vi "精度表.vi"() -> (2 "精度":i32[](array[numeric]), 3 "参数":string[](array[string]))   [LabVIEW 2016, in "数据查询.lvlib"]
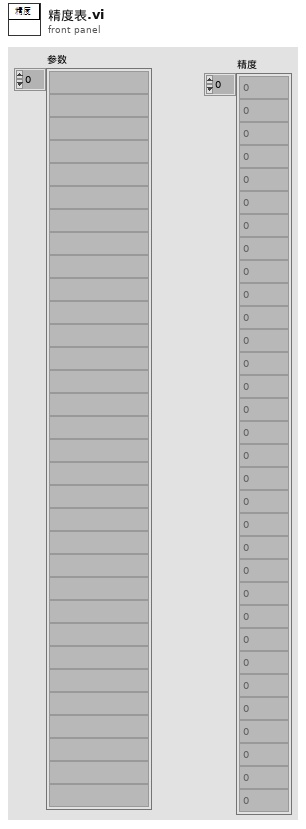
[diagram p1: front panel]
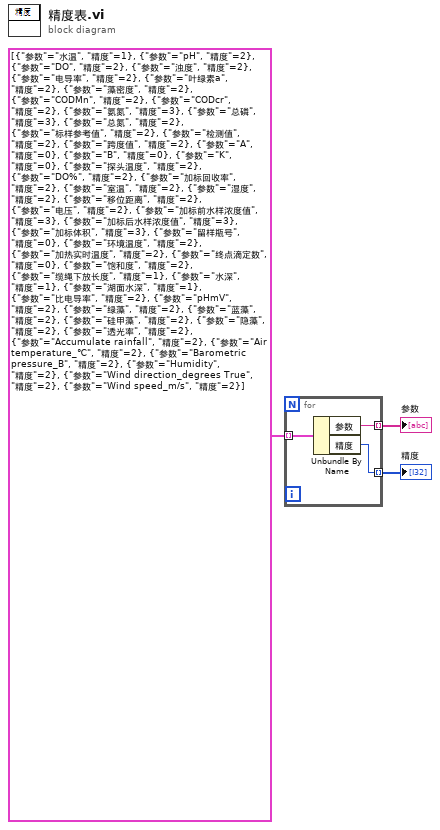
[diagram p0: block diagram]
diagram:
  n1 = for {
    tunnel: cluster{"参数":string, "精度":i32}[] [{"参数"="水温", "精度"=1}, {"参数"="pH", "精度"=2}, {"参数"="DO", "精度"=2}, {"参数"="浊度", "精度"=2}, {"参数"="电导率", "精度"=2}, {"参数"="叶绿素a", "精度"=2}, {"参数"="藻密度", "精度"=2}, {"参数"="CODMn", "精度"=2}, {"参数"="CODcr", "精度"=2}, {"参数"="氨氮", "精度"=3}, {"参数"="总磷", "精度"=3}, {"参数"="总氮", "精度"=2}, {"参数"="标样参考值", "精度"=2}, {"参数"="检测值", "精度"=2}, {"参数"="跨度值", "精度"=2}, {"参数"="A", "精度"=0}, {"参数"="B", "精度"=0}, {"参数"="K", "精度"=0}, {"参数"="探头温度", "精度"=2}, {"参数"="DO%", "精度"=2}, {"参数"="加标回收率", "精度"=2}, {"参数"="室温", "精度"=2}, {"参数"="湿度", "精度"=2}, {"参数"="移位距离", "精度"=2}, {"参数"="电压", "精度"=2}, {"参数"="加标前水样浓度值", "精度"=3}, {"参数"="加标后水样浓度值", "精度"=3}, {"参数"="加标体积", "精度"=3}, {"参数"="留样瓶号", "精度"=0}, {"参数"="环境温度", "精度"=2}, {"参数"="加热实时温度", "精度"=2}, {"参数"="终点滴定数", "精度"=0}, {"参数"="饱和度", "精度"=2}, {"参数"="缆绳下放长度", "精度"=1}, {"参数"="水深", "精度"=1}, {"参数"="湖面水深", "精度"=1}, {"参数"="比电导率", "精度"=2}, {"参数"="pHmV", "精度"=2}, {"参数"="绿藻", "精度"=2}, {"参数"="蓝藻", "精度"=2}, {"参数"="硅甲藻", "精度"=2}, {"参数"="隐藻", "精度"=2}, {"参数"="透光率", "精度"=2}, {"参数"="Accumulate rainfall", "精度"=2}, {"参数"="Air temperature_℃", "精度"=2}, {"参数"="Barometric pressure_B", "精度"=2}, {"参数"="Humidity", "精度"=2}, {"参数"="Wind direction_degrees True", "精度"=2}, {"参数"="Wind speed_m/s", "精度"=2}] ("数组") -> [w6] mode=indexing
    tunnel: [w5] -> w2 mode=indexing
    tunnel: [w4] -> w1 mode=indexing
    n2 = Unbundle By Name(w6) -> ("参数"=w5:string, "精度"=w4:i32)
  }
  "参数" <- w2
  "精度" <- w1
